vi "RawToTemp.vi"(0 "reference in":refnum<class "BME280.lvclass">, 2 "T_ADC":dbl, 5 "error in (no error)":errorcluster) -> (14 "reference out":refnum<class "BME280.lvclass">, 16 "T":dbl, 19 "error out":errorcluster)   [LabVIEW 2014, in "BME280.lvclass"]
uses:
  BME280.lvclass
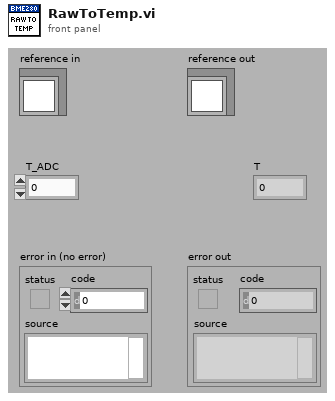
[diagram p1: front panel]
types:
  T1 = typedef "BME280.lvclass/ObjectAttributes.ctl" = cluster{"I2C Slave Address":u8, "TrimmingParameters":T2, "t_fine":i32}
  T2 = typedef "BME280.lvclass/TrimmingParameters.ctl" = cluster{"dig_T1":u16, "dig_T2":i16, "dig_T3":i16, "dig_P1":u16, "dig_P2":i16, "dig_P3":i16, "dig_P4":i16, "dig_P5":i16, "dig_P6":i16, "dig_P7":i16, "dig_P8":i16, "dig_P9":i16, "dig_H1":u8, "dig_H2":i16, "dig_H3":u8, "dig_H4":i16, "dig_H5":i16, "dig_H6":i8}
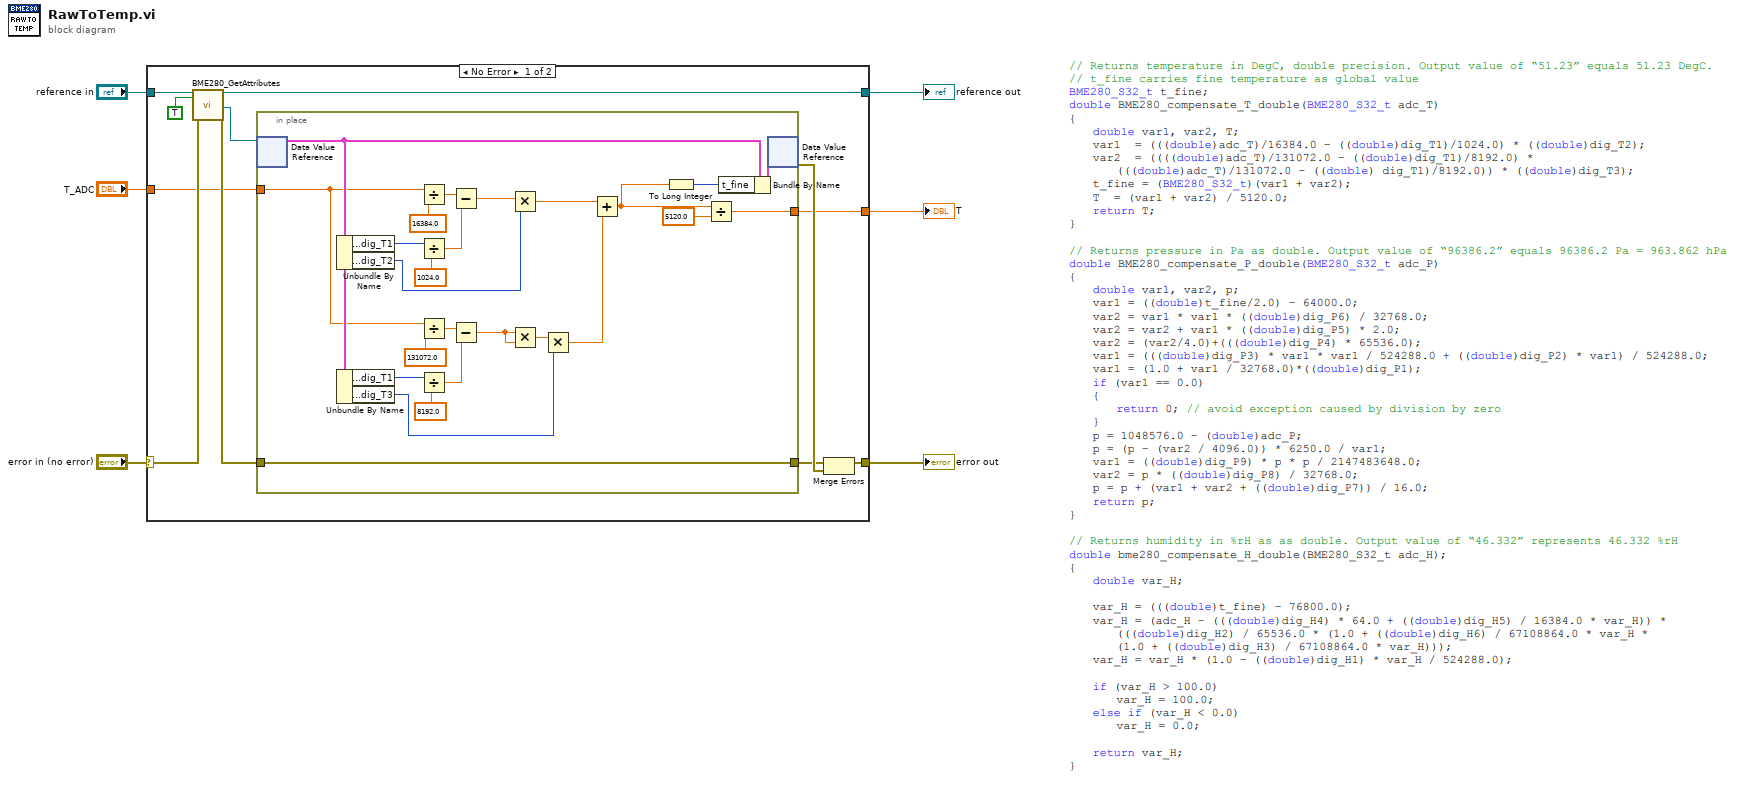
[diagram p0: block diagram]
diagram:
  n1 = case shown="No Error" "error in (no error)" {
    selector: "error in (no error)" -> [w14 w44]
    tunnel: [w16 w44] -> w5
    tunnel: [w12 w43] -> w3
    tunnel: "reference in" -> [w15 w43]
    tunnel: "T_ADC" -> [w8 _]
    tunnel: [w7 _] -> w1
    frame No Error {
      n2 = call "BME280_GetAttributes.vi"("reference in"=w15, "OnlyGetDvrReference(False)"=TRUE, "error in (no error)"=w14) -> ("reference out"=w12:refnum<class "BME280.lvclass">, "DataRef"=w13:refnum<data-value>, "error out"=w10:errorcluster)  [unwired: 13 in, 1 out]
      n3 = in-place {
        in-place-border: w10 -> [w41]
        in-place-border: [w41] -> w9
        in-place-border: w8 -> [w27]
        in-place-border: [w22] -> w7
        n4 = in-place-dvr #1(w13) -> (w28:T1)  [unwired: 1 out]
        n5 = Unbundle By Name(w28) -> ("TrimmingParameters.dig_T1"=w37:u16, "TrimmingParameters.dig_T2"=w34:i16)
        n6 = Unbundle By Name(w28) -> ("TrimmingParameters.dig_T1"=w32:u16, "TrimmingParameters.dig_T3"=w19:i16)
        n7 = Divide(x=w27, y=16384.0) -> (x/y=w39:dbl)
        n8 = Divide(x=w37, y=1024.0) -> (x/y=w36:dbl)
        n9 = Divide(x=w27, y=131072.0) -> (x/y=w30:dbl)
        n10 = Divide(x=w32, y=8192.0) -> (x/y=w33:dbl)
        n11 = Subtract(x=w39, y=w36) -> (x-y=w35:dbl)
        n12 = Subtract(x=w30, y=w33) -> (x-y=w21:dbl)
        n13 = Multiply(x=w35, y=w34) -> (x*y=w26:dbl)
        n14 = Multiply(x=w21, y=w21) -> (x*y=w20:dbl)
        n15 = Multiply(x=w20, y=w19) -> (x*y=w18:dbl)
        n16 = Add(x=w26, y=w18) -> (x+y=w24:dbl)
        n17 = To Long Integer(number=w24) -> (32bit integer=w25:i32)
        n18 = Divide(x=w24, y=5120.0) -> (x/y=w22:dbl)
        n19 = Bundle By Name(cluster=w28, "t_fine"=w25) -> (w42:T1)
        n20 = in-place-dvr #1(w42) -> (w17:errorcluster)  [unwired: 1 out]
      }
      n21 = Merge Errors(w9, w17) -> (w16:errorcluster)
    }
    frame Error {
    }
  }
  "error out" <- w5
  "reference out" <- w3
  "T" <- w1
